vi "Create from SQL Record.vi"(8 "error in (no error)":errorcluster, 11 "MySQL Record":variant[](array[variant])) -> (0 "error out":errorcluster, 3 "Credit Record out":refnum<class "Credit Transaction.lvclass">)   [LabVIEW 2018, in "Credit Transaction.lvclass"]
uses:
  Credit Transaction.lvclass
  C:/Users/Jeff Tipps/Documents/Filthy-Lucre-Budgetizer/source/support/classes/Transaction/Transaction.lvclass
  Transaction/Transaction.lvclass
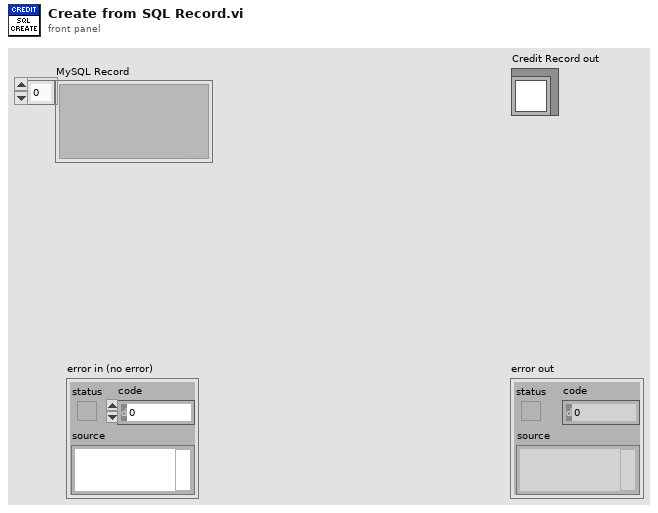
[diagram p1: front panel]
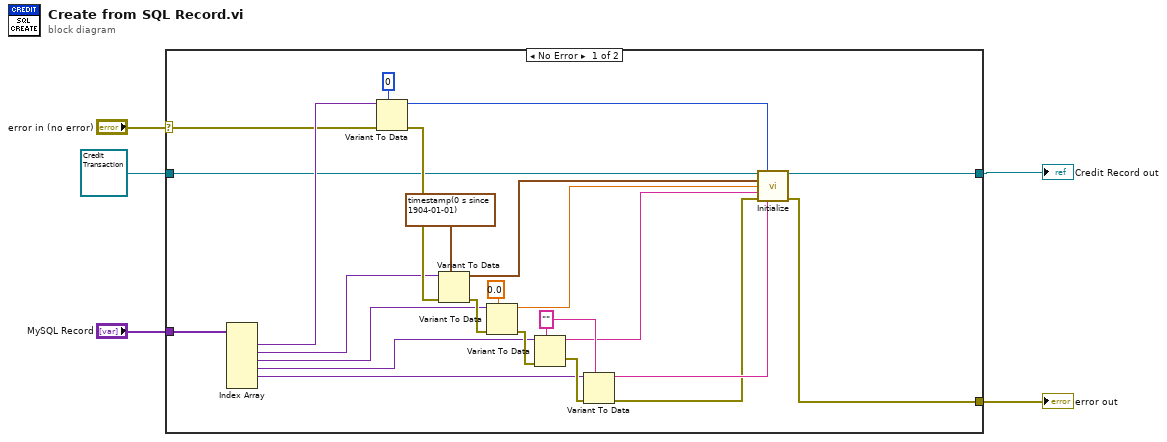
[diagram p0: block diagram]
diagram:
  n1 = case shown="No Error" "error in (no error)" {
    selector: "error in (no error)" -> [w19 w31]
    tunnel: [w6 w30] -> w2
    tunnel: [w13 w31] -> w5
    tunnel: refnum<class "Credit Transaction.lvclass"> refnum ("Credit Record in") -> [w16 w30]
    tunnel: "MySQL Record" -> [w18 _]
    frame No Error {
      w10 = ""
      n2 = Index Array(array=w18) -> (element #1=w25:variant, element #2=w17:variant, element #3=w24:variant, element #4=w23:variant, element #5=w22:variant)  [unwired: 6 in, 1 out]
      n3 = Variant To Data(error in=w19, type=0 ("id"), Variant=w25) -> (data=w15:i32, error out=w29:errorcluster)
      n4 = Variant To Data(error in=w29, type=timestamp(0 s since 1904-01-01), Variant=w17) -> (data=w14:timestamp, error out=w26:errorcluster)
      n5 = Variant To Data(error in=w26, type=0.0 ("Amount"), Variant=w24) -> (data=w11:dbl, error out=w27:errorcluster)
      n6 = Variant To Data(error in=w27, type=w10, Variant=w23) -> (data=w9:string, error out=w28:errorcluster)
      n7 = Variant To Data(error in=w28, type=w10, Variant=w22) -> (data=w8:string, error out=w7:errorcluster)
      n8 = call "Initialize.vi"("Transaction in"=w16, "ID"=w15, "Date"=w14, "Amount"=w11, "Description"=w9, "error in (no error)"=w7, "Category"=w8) -> ("Transaction out"=w6:refnum<class "Credit Transaction.lvclass">, "error out"=w13:errorcluster)  [unwired: 7 in]
    }
    frame Error {
    }
  }
  "error out" <- w5
  "Credit Record out" <- w2
